vi "Get Protocol Classes List.vi"(8 "error in (no error)":errorcluster) -> (0 "error out":errorcluster, 3 "Class Lookup":variant)   [LabVIEW 2018, in "Instrument Addon Scripting API.lvlib"]
uses:
  Instrument Addon Scripting API.lvlib
  <vilib>/Utility/sysdir.llb/System Directory Type.ctl
  <vilib>/Utility/LVLibp/NI_PackedLibraryUtility.lvlib
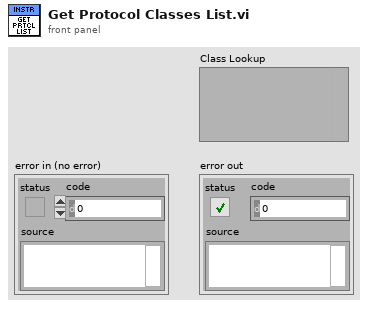
[diagram p1: front panel]
types:
  T1 = typedef "System Directory Type.ctl" = i32
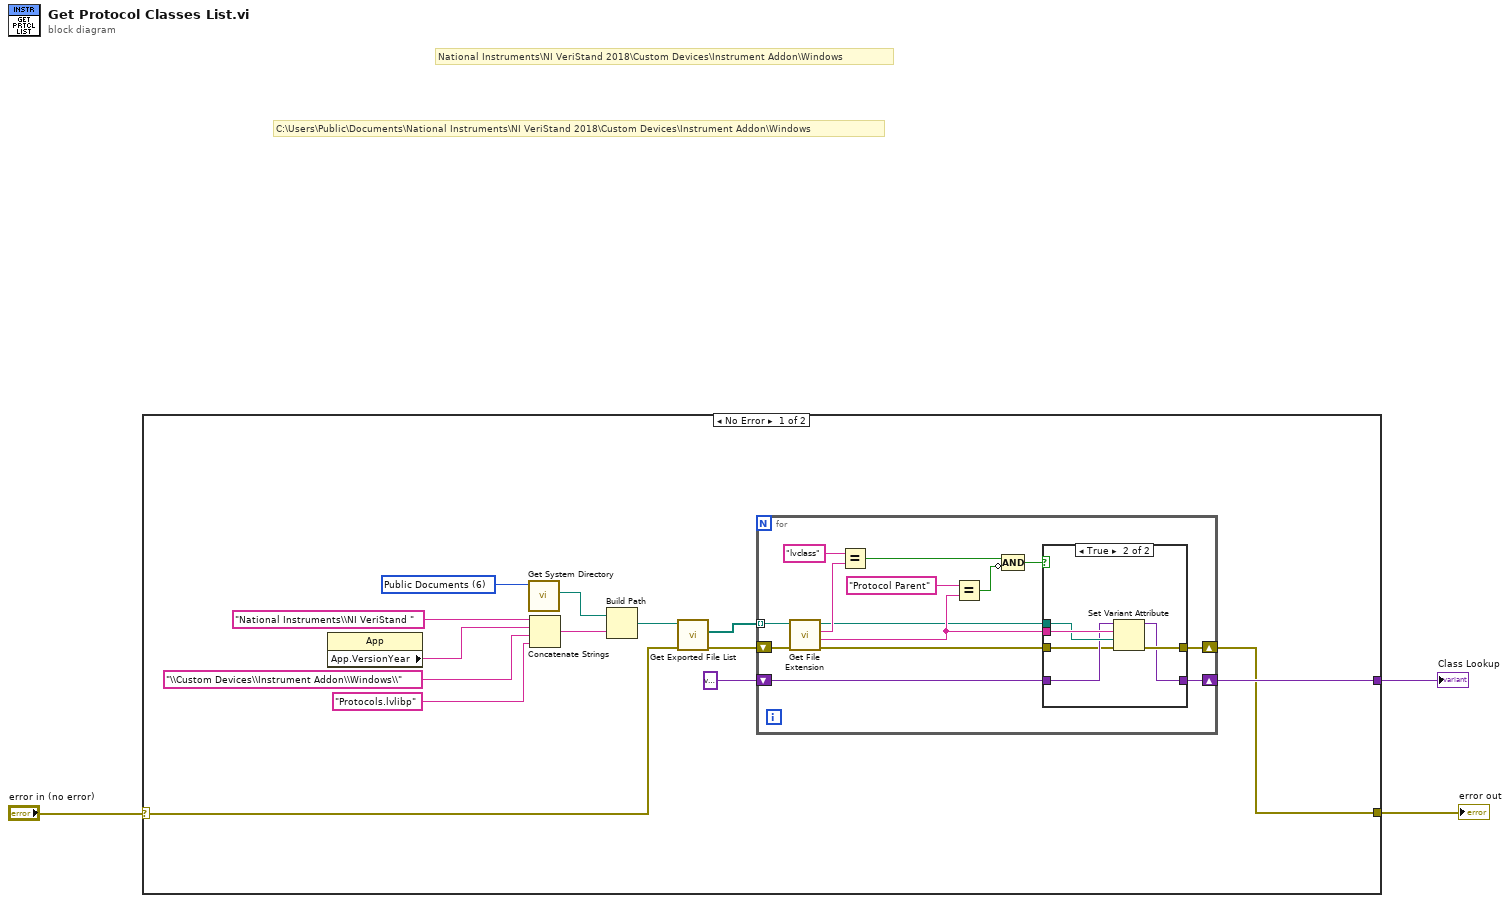
[diagram p0: block diagram]
diagram:
  # "National Instruments\\NI VeriStand 2018\\Custom Devices\\Instrument Addon\\Windows"
  # "C:\\Users\\Public\\Documents\\National Instruments\\NI VeriStand 2018\\Custom Devices\\Instrument Addon\\Windows"
  n1 = case shown="No Error" "error in (no error)" {
    selector: "error in (no error)" -> [w4 w40]
    tunnel: [w17 _] -> w3
    tunnel: [w16 w40] -> w2
    frame No Error {
      w15 = T1 6 items=["User Home"=0, "User Desktop"=1, "User Documents"=2, "User Application Data"=3, "User Preferences"=4, "User Temporary"=5, "Public Documents"=6, "Public Application Data"=7, "Public Preferences"=8, "Public Cache"=13, "System Core Libraries"=9, "System Installed Libraries"=10, "Application Files"=11, "Boot Volume Root"=12] ("system directory type")
      n2 = property class="App"() -> ("App.VersionYear"=w11:string)  [unwired: 2 in, 2 out]
      n3 = call <vilib>:"Get System Directory.vi"("system directory type"=w15) -> ("system directory"=w14:path)  [unwired: 10 in]
      n4 = Concatenate Strings("National Instruments\\NI VeriStand " ("string"), w11, "\\Custom Devices\\Instrument Addon\\Windows\\" ("string"), "Protocols.lvlibp" ("name or relative path")) -> (w13:string)
      n5 = Build Path(base path=w14, name or relative path=w13) -> (appended path=w5:path)
      n6 = call <vilib>:"Get Exported File List.vi"("error in (no error)"=w4, "packed library path"=w5) -> ("error out"=w7:errorcluster, "paths"=w6:path[])  [unwired: 7 in, 1 out]
      n7 = for {
        tunnel: w6 -> [w26] mode=indexing
        shift-right: [w20] -> w16
        shift-left: w7 -> [w27]
        shift-right: [w19] -> w17
        shift-left: variant ("variant") -> [w22]
        n8 = call <vilib>:"Get File Extension.vi"("error in (no error)"=w27, "file"=w26) -> ("error out"=w21:errorcluster, "filename without extension"=w24:string, "lowercase file extension"=w28:string, "dup file"=w23:path)  [unwired: 5 in, 1 out]
        n9 = Equal?(x="lvclass" ("string"), y=w28) -> (x = y?=w30:bool)
        n10 = Equal?(x="Protocol Parent", y=w24) -> (x = y?=w25:bool)
        n11 = Compound Arithmetic op=AND(w30, invert w25) -> (w18:bool)
        n12 = case shown="True" w18 {
          tunnel: w24 -> [_ w39]
          tunnel: w23 -> [_ w38]
          tunnel: w22 -> [w32 w37]
          tunnel: w21 -> [w33 w36]
          tunnel: [w33 w35] -> w20
          tunnel: [w32 w34] -> w19
          frame False {
          }
          frame True {
            n13 = Set Variant Attribute(Variant=w37, name=w39, value=w38, error in=w36) -> (Variant out=w34:variant, error out=w35:errorcluster)  [unwired: 1 out]
          }
        }
      }
    }
    frame Error {
    }
  }
  "Class Lookup" <- w3
  "error out" <- w2
